vi "Strain_w_User_Feedback_Solution.vi"() -> ()   [LabVIEW 2013]
uses:
  <vilib>/DAQmx/read.llb/DAQmx Read (Analog Wfm 1Chan NSamp).vi
  <vilib>/DAQmx/write.llb/DAQmx Write (Digital 1D Bool 1Chan 1Samp).vi
  <vilib>/DAQmx/create/channels.llb/DAQmx Create Channel (AI-Strain-Strain Gage).vi
  <vilib>/DAQmx/create/channels.llb/DAQmx Create Channel (DO-Digital Output).vi
  <vilib>/DAQmx/configure/timing.llb/DAQmx Timing (Sample Clock).vi
  <vilib>/DAQmx/miscellaneous.llb/DAQmx Fill In Error Info.vi
panel:
  in  "LED Channels":tag="Digital_out/port0/line0:7"
  in  "Samples Per Channel":i32=1000
  in  "Strain Sample Rate":dbl=10000.0
  in  "DAQmx Physical Channel":tag="Strain/ai0"
  in  "Number of LEDs":i32=8
  in  "Stop Button":bool
  in  "Range Low":dbl
  in  "Range High":dbl=0.001
  out "LED Out":bool[](array[boolean])
  out "Strain Chart":waveform(dbl)(graph)={"t0"=timestamp(3432646805.8013763 s since 1904-01-01), "dt"=9.999999999999999e-05, "Y"=[-0.00021477239091112946, -0.00021657267011829324, -0.00021557095914165154, -0.0002130071302958166, -0.0002147093459964931, -0.00021465330606569694, -0.00021571806367655234, -0.0002155079143277281, -0.0002147793959011538, -0.00021528375492494025, -0.0002148424408069557, -0.00021577410348798507, -0.00021435209133003415, -0.0002131892606476988, -0.0002139247863936575, -0.000211760236104557, -0.00021395280640067584, -0.00021340641598052517, -0.00021325931076536907, -0.0002163555161608963, -0.00021585115821844725, -0.00021472335597821053, -0.00021529075990779886, -0.00021370062628097, -0.00021367961126525205, -0.00021298611525094477, -0.0002141419414069692, -0.0002150385804630476, -0.00021440813129459767, -0.000213959811402185, -0.00021482843082857575, -0.00021589318806642047, -0.00021562699896957526, -0.00021491949568102698, -0.00021710504716311428, -0.0002149965505432208, -0.0002156129890131833, -0.0002132312907194789, -0.00021400884641000078, -0.00021493350565685474, -0.00021458325614336725, -0.00021366560125428264, -0.0002144991962236144, -0.0002158651681681643, -0.00021480041087063788, -0.00021342743100772794, -0.00021456924615772337, -0.00021346946105948314, -0.00021519269013884568, -0.00021440813129459767, -0.00021395280640067584, -0.00021368661627058953, -0.00021579511841565268, -0.0002150315754766552, -0.00021564100892557456, -0.00021560598403484008, -0.00021615237205083515, -0.00021412793140895706, -0.0002149615256073324, -0.00021431006135248876, -0.00021615937702152186, -0.00021485645078494301, -0.00021334337089361612, -0.0002151366502622343, -0.0002147093459964931, -0.00021610333725327976, -0.0002150385804630476, -0.00021424701637954479, -0.0002146463010739057, -0.00021505259043553792, -0.00021493350565685474, -0.00021632049132022367, -0.00021340641598052517, -0.00021362357121901854, -0.00021519269013884568, -0.00021362357121901854, -0.00021419097639691965, -0.00021430305635588762, -0.00021511563530688535, -0.0002142750363685015, -0.00021372164129580443, -0.00021454823117852137, -0.00021446417125287886, -0.00021387575137759622, -0.00021466031105739, -0.00021568303879121667, -0.00021402986141187797, -0.00021487746575118776, -0.00021514365524715427, -0.00021399483640825853, -0.00021411392141055228, -0.00021594922785822106, -0.0002135605261594965, -0.00021485645078494301, -0.00021406488641304342, -0.00021592821293703202, -0.00021505259043553792], "attributes"=variant("NI_ChannelName"=variant(string "Strain/ai0"), "NI_UnitDescription"=variant(string "Strain"))}
  # "LED Configuration"
  # "Quarter Bridge Diagram"
  # "Strain Configuration"
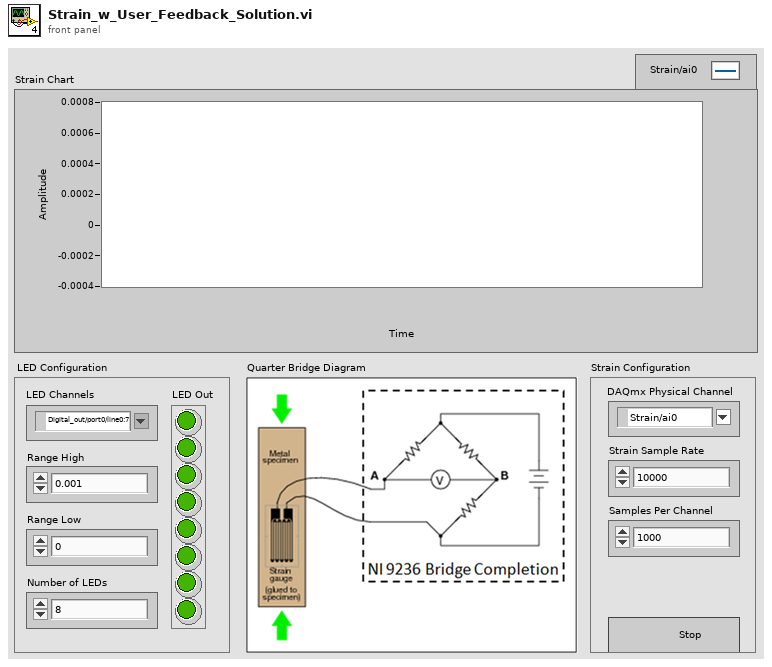
[diagram p1: front panel]
types:
  T1 = cluster{"gage factor":dbl, "nominal gage resistance":dbl, "poisson ratio":dbl}
  T2 = cluster{"strain configuration":i32, "lead wire resistance":dbl, "initial bridge voltage":dbl, "voltage excitation source":i32, "voltage excitation value":dbl}
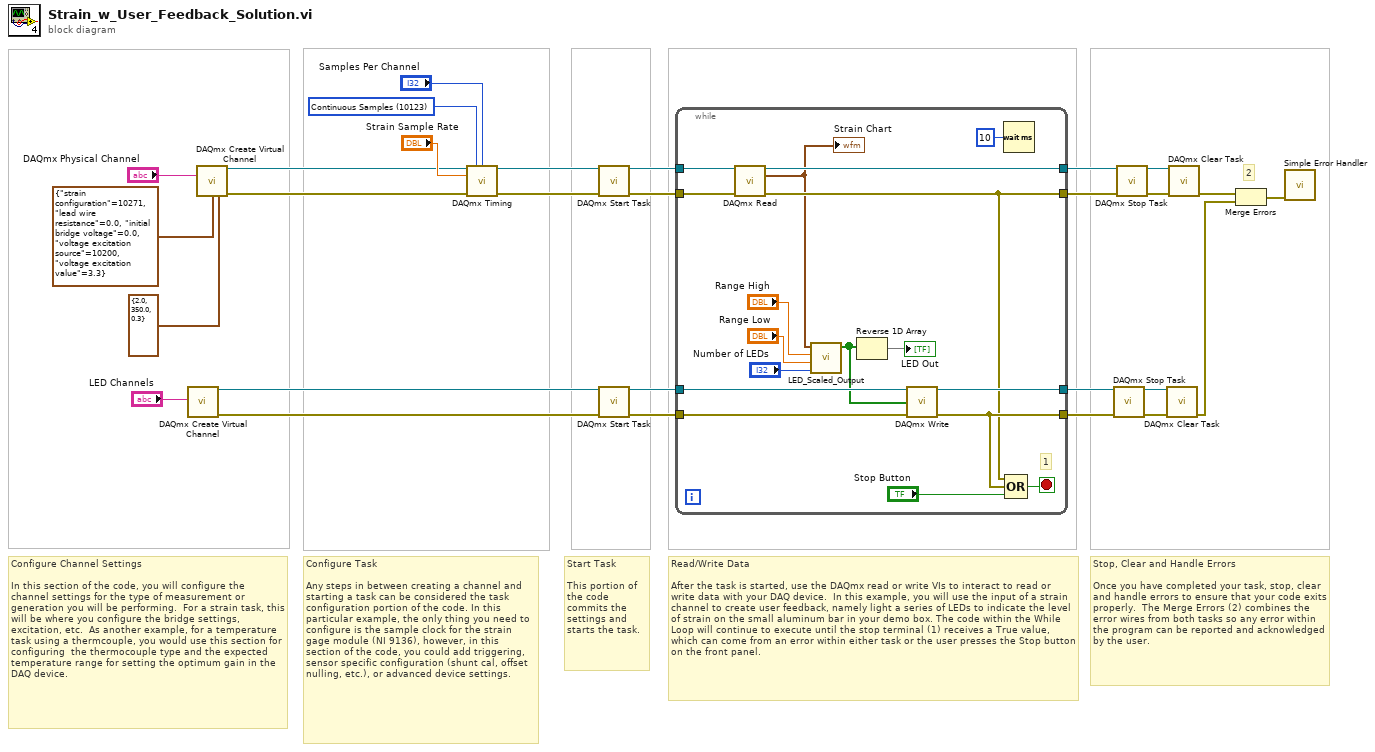
[diagram p0: block diagram]
diagram:
  w1 = 10123 items=["Finite Samples"=10178, "Continuous Samples"=10123, "Hardware Timed Single Point"=12522] ("sample mode")
  # "2"
  # "Stop, Clear and Handle Errors\n\nOnce you have completed your task, stop, clear and handle errors to ensure that your code exits properly.  The Merge Errors (2) combines the error wires from both tasks so any error within the program can be reported and acknowledged by the user."
  # "Read/Write Data\n\nAfter the task is started, use the DAQmx read or write VIs to interact to read or write data with your DAQ device.  In this example, you will use the input of a strain channel to create user feedback, namely light a series of LEDs to indicate the level of strain on the small aluminum bar in your demo box. The code within the While Loop will continue to execute until the stop terminal (1) receives a True value, which can come from an error within either task or the user presses the Stop button on the front panel."
  # "Start Task\n\nThis portion of the code commits the settings and starts the task."
  # "Configure Task\n\nAny steps in between creating a channel and starting a task can be considered the task configuration portion of the code. In this particular example, the only thing you need to configure is the sample clock for the strain gage module (NI 9136), however, in this section of the code, you could add triggering, sensor specific configuration (shunt cal, offset nulling, etc.), or advanced device settings."
  # "Configure Channel Settings\n\nIn this section of the code, you will configure the channel settings for the type of measurement or generation you will be performing.  For a strain task, this will be where you configure the bridge settings, excitation, etc.  As another example, for a temperature task using a thermcouple, you would use this section for configuring  the thermocouple type and the expected temperature range for setting the optimum gain in the DAQ device."
  n1 = call-poly <vilib>:"DAQmx Create Virtual Channel.vi"("lines"="LED Channels") -> ("task out"=w18:refnum<k21>, "error out"=w17:errorcluster)  [unwired: 13 in]
  n2 = call-poly <vilib>:"DAQmx Create Virtual Channel.vi"("physical channels"="DAQmx Physical Channel", "bridge information"=T2 {"strain configuration"=10271, "lead wire resistance"=0.0, "initial bridge voltage"=0.0, "voltage excitation source"=10200, "voltage excitation value"=3.3}, "strain gage information"=T1 {"gage factor"=2.0, "nominal gage resistance"=350.0, "poisson ratio"=0.3}) -> ("task out"=w27:refnum<k21>, "error out"=w22:errorcluster)  [unwired: 11 in]
  n3 = call-poly <vilib>:"DAQmx Timing.vi"("task/channels in"=w27, "sample mode"=w1, "samples per channel"="Samples Per Channel", "rate"="Strain Sample Rate", "error in"=w22) -> ("task out"=w26:refnum<k21>, "error out"=w4:errorcluster)  [unwired: 9 in]
  n4 = call <vilib>:"DAQmx Start Task.vi"("task/channels in"=w26, "error in"=w4) -> ("task out"=w25:refnum<k21>, "error out"=w3:errorcluster)  [unwired: 12 in]
  n5 = call <vilib>:"DAQmx Start Task.vi"("task/channels in"=w18, "error in"=w17) -> ("task out"=w16:refnum<k21>, "error out"=w15:errorcluster)  [unwired: 12 in]
  n6 = while {
    tunnel: w25 -> [w45]
    tunnel: [w44] -> w24
    tunnel: w16 -> [w41]
    tunnel: w15 -> [w40]
    tunnel: [w35] -> w14
    tunnel: [w39] -> w13
    tunnel: [w34] -> w12
    tunnel: w3 -> [w32]
    stop <- w43 stop-if-true
    # "1"
    n7 = call-poly <vilib>:"DAQmx Read.vi"("task/channels in"=w45, "error in"=w32) -> ("task out"=w44:refnum<k21>, "data"=w33:waveform(dbl), "error out"=w34:errorcluster)  [unwired: 11 in]
    "Strain Chart" <- w33
    n8 = call "LED_Scaled_Output.vi"("Number of LEDs"="Number of LEDs", "Range Bottom"="Range Low", "Range Top"="Range High", "Sensor Input"=w33) -> ("Output (bool)"=w30:bool[])  [unwired: 4 in, 3 out]
    n9 = Reverse 1D Array(array=w30) -> (reversed array=→"LED Out":bool[])
    n10 = call-poly <vilib>:"DAQmx Write.vi"("task/channels in"=w41, "data"=w30, "error in"=w40) -> ("task out"=w39:refnum<k21>, "error out"=w35:errorcluster)  [unwired: 10 in, 1 out]
    n11 = Wait (ms)(milliseconds to wait=u32 10) -> ()  [unwired: 1 out]
    n12 = Compound Arithmetic op=OR(w34, w35, "Stop Button") -> (w43:bool)
  }
  n13 = call <vilib>:"DAQmx Stop Task.vi"("task/channels in"=w13, "error in"=w14) -> ("task out"=w10:refnum<k21>, "error out"=w11:errorcluster)  [unwired: 12 in]
  n14 = call <vilib>:"DAQmx Stop Task.vi"("task/channels in"=w24, "error in"=w12) -> ("task out"=w23:refnum<k21>, "error out"=w6:errorcluster)  [unwired: 12 in]
  n15 = call <vilib>:"DAQmx Clear Task.vi"("task in"=w10, "error in"=w11) -> ("error out"=w9:errorcluster)  [unwired: 13 in]
  n16 = call <vilib>:"DAQmx Clear Task.vi"("task in"=w23, "error in"=w6) -> ("error out"=w7:errorcluster)  [unwired: 13 in]
  n17 = Merge Errors(w7, w9) -> (w8:errorcluster)
  n18 = call <vilib>:"Simple Error Handler.vi"("error in (no error)"=w8) -> ()  [unwired: 4 in, 5 out]
